vi "Create.vi"(8 "error in (no error)":errorcluster, 10 "Player name":string) -> (0 "error out":errorcluster, 3 "Player.lvclass":refnum<class "Player.lvclass">)   [LabVIEW 2016, in "Player.lvclass"]
uses:
  Player.lvclass
  Player.lvclass/Player.ctl
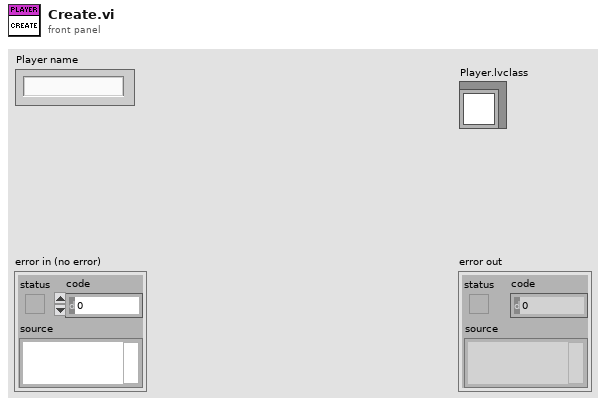
[diagram p1: front panel]
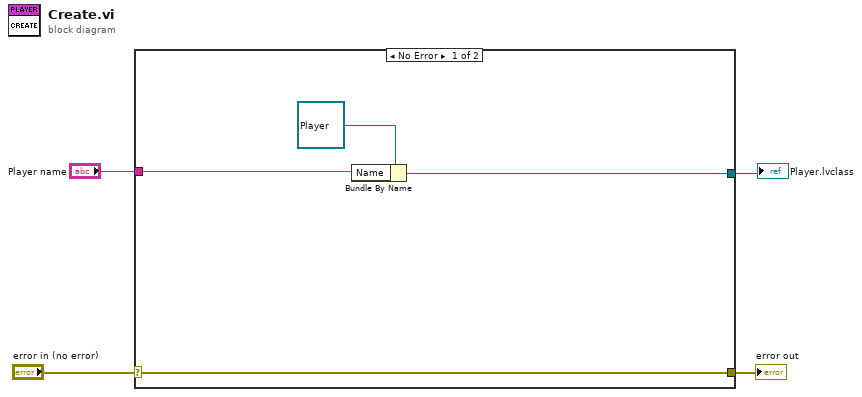
[diagram p0: block diagram]
diagram:
  n1 = case shown="No Error" "error in (no error)" {
    selector: "error in (no error)" -> [w8 w9]
    tunnel: [w8 w9] -> w3
    tunnel: "Player name" -> [w6 _]
    tunnel: [w5 _] -> w1
    frame No Error {
      n2 = Bundle By Name(cluster=refnum<class "Player.lvclass"> refnum ("Player.lvclass 2"), "Name"=w6) -> (w5:refnum<class "Player.lvclass">)
    }
    frame Error {
    }
  }
  "error out" <- w3
  "Player.lvclass" <- w1
